vi "X509_get_subject_name.vi"(8 "error in (no error)":errorcluster, 11 "X509-Cert in":refnum<class "X509-Cert.lvclass">) -> (0 "error out":errorcluster, 2 "subject name":string, 3 "X509-Cert out":refnum<class "X509-Cert.lvclass">)   [LabVIEW 2013, in "OpenSSL Socket.lvlib" / "X509-Cert.lvclass"]
uses:
  X509-Cert.lvclass
  SSL-Lib/SSL-Lib.lvclass/SSL-Lib.ctl
  X509-Cert.lvclass/X509-Cert.ctl
  SSL-Lib/Read Crypto Library Path.vi
  Read Handle.vi
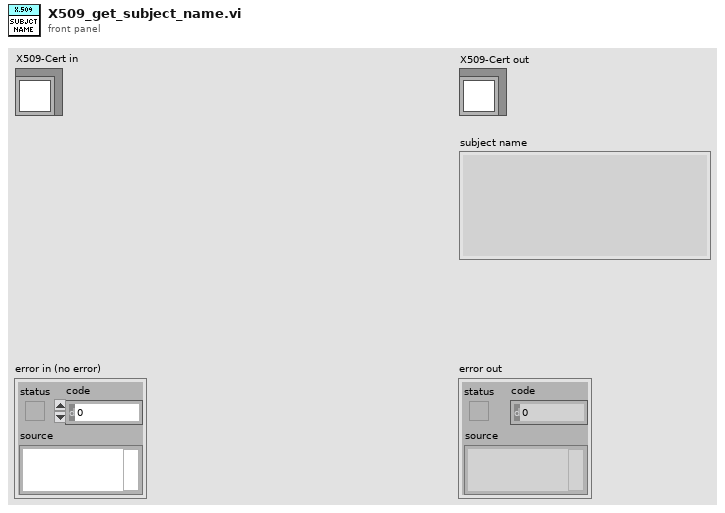
[diagram p1: front panel]
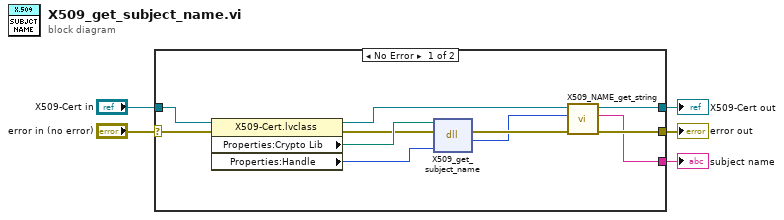
[diagram p0: block diagram]
diagram:
  n1 = case shown="No Error" "error in (no error)" {
    selector: "error in (no error)" -> [w15 w18]
    tunnel: [w8 w18] -> w4
    tunnel: "X509-Cert in" -> [w16 w17]
    tunnel: [w7 _] -> w2
    tunnel: [w9 w17] -> w1
    frame No Error {
      n2 = property class="X509-Cert.lvclass"(reference=w16, error in=w15) -> (reference out=w10:refnum<class "X509-Cert.lvclass">, error out=w12:errorcluster, "Properties:Crypto Lib"=w13:path, "Properties:Handle"=w14:u64)
      n3 = dll-call lib="C:/Program Files (x86)/National Instruments/Shared/nissl/NIlibeay32.dll" fn="X509_get_subject_name"(path in=w13, error in=w12, "X509"=w14) -> (error out=w11:errorcluster, "return type"=w6:u64)  [unwired: 2 in, 1 out]
      n4 = call "X509_NAME_get_string.vi"("error in (no error)"=w11, "X509_Name"=w6, "X509-Cert in"=w10) -> ("error out"=w8:errorcluster, "X509 Name String"=w7:string, "X509-Cert out"=w9:refnum<class "X509-Cert.lvclass">)  [unwired: 6 in]
    }
    frame Error {
    }
  }
  "error out" <- w4
  "subject name" <- w2
  "X509-Cert out" <- w1
